vi "Drive Towards Gap.vi"(5 "max forward velocity (m/s)":dbl, 7 "max angular velocity (rad/s)":dbl=1.0, 8 "error in (no error)":errorcluster, 11 "gap":T1) -> (0 "error out":errorcluster, 2 "steering frame velocity":dbl[](array[numeric]))   [LabVIEW 2013]
doc: "Sets the steering frame velocity so that the robot moves towards the gap."
uses:
  <vilib>/robotics/Obstacle Avoidance/Simple Vector Field Histogram/Gap Description.ctl
  <vilib>/robotics/Obstacle Avoidance/Simple Vector Field Histogram/NI_Robotics_Simple Vector Field Histogram.lvlib
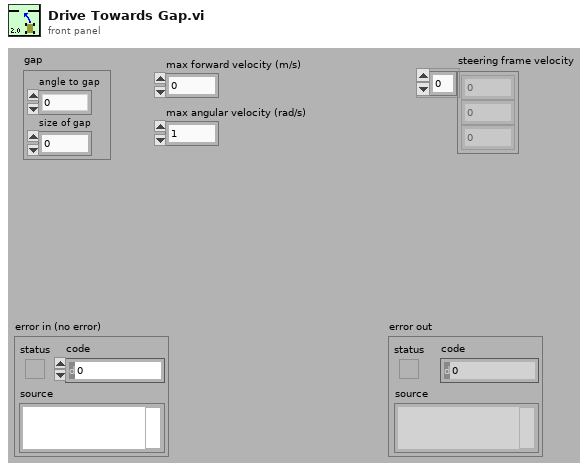
[diagram p1: front panel]
types:
  T1 = typedef "NI_Robotics_Simple Vector Field Histogram.lvlib/Gap Description.ctl" = cluster{"angle to gap":dbl, "size of gap":dbl}
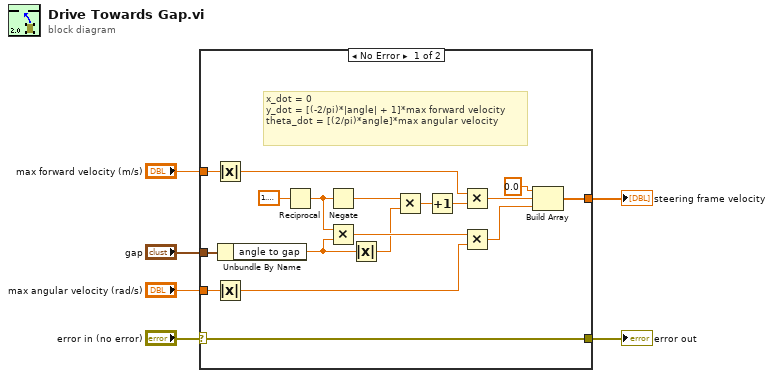
[diagram p0: block diagram]
diagram:
  n1 = case shown="No Error" "error in (no error)" {
    selector: "error in (no error)" -> [w23 w25]
    tunnel: "gap" -> [w24 _]
    tunnel: [w23 w25] -> w4
    tunnel: "max forward velocity (m/s)" -> [w18 _]
    tunnel: "max angular velocity (rad/s)" -> [w14 _]
    tunnel: [w10 _] -> w1
    frame No Error {
      # "x_dot = 0\ny_dot = [(-2/pi)*|angle| + 1]*max forward velocity\ntheta_dot = [(2/pi)*angle]*max angular velocity"
      n2 = Absolute Value(x=w18) -> (abs(x)=w9:dbl)
      n3 = Absolute Value(x=w14) -> (abs(x)=w8:dbl)
      n4 = Unbundle By Name(w24) -> ("angle to gap"=w16:dbl)
      n5 = Reciprocal(x=1.5707963267948966) -> (1/x=w17:dbl)
      n6 = Negate(x=w17) -> (-x=w21:dbl)
      n7 = Multiply(x=w17, y=w16) -> (x*y=w15:dbl)
      n8 = Absolute Value(x=w16) -> (abs(x)=w7:dbl)
      n9 = Multiply(x=w21, y=w7) -> (x*y=w20:dbl)
      n10 = Increment(x=w20) -> (x+1=w19:dbl)
      n11 = Multiply(x=w9, y=w19) -> (x*y=w13:dbl)
      n12 = Multiply(x=w15, y=w8) -> (x*y=w12:dbl)
      n13 = Build Array(0.0 ("element"), w13, w12) -> (w10:dbl[])
    }
    frame Error {
    }
  }
  "error out" <- w4
  "steering frame velocity" <- w1
